vi "ep_Check Time Domain Parameters.vi"(5 "actual ranges [%]":dbl[](array[numeric]), 7 "ranges to calibrate [%]":dbl[](array[numeric]), 8 "error in (no error)":errorcluster, 9 "gains":dbl[][](array[numeric]), 10 "offsets":dbl[](array[numeric]), 11 "waveforms in":waveform(dbl)[](array[waveform])) -> (0 "error out":errorcluster)   [LabVIEW 2014, in "NI_EP_Power Quality.lvlib"]
uses:
  <vilib>/addons/Electrical Power/PQ/NI_EP_Power Quality.lvlib
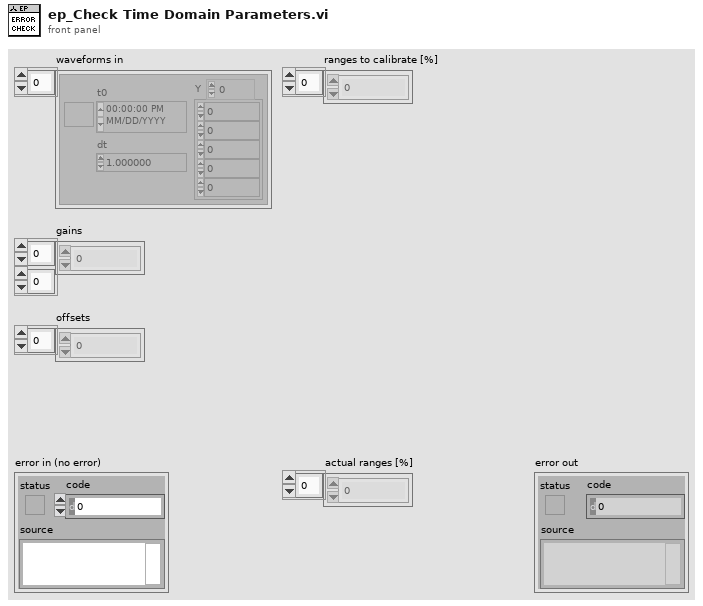
[diagram p1: front panel]
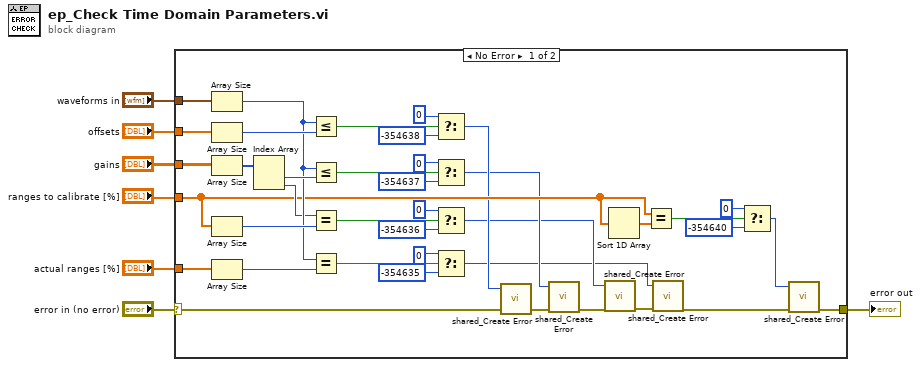
[diagram p0: block diagram]
diagram:
  n1 = case shown="No Error" "error in (no error)" {
    selector: "error in (no error)" -> [w8 w47]
    tunnel: "waveforms in" -> [w45 _]
    tunnel: "offsets" -> [w44 _]
    tunnel: "actual ranges [%]" -> [w43 _]
    tunnel: "gains" -> [w40 _]
    tunnel: "ranges to calibrate [%]" -> [w35 _]
    tunnel: [w9 w47] -> w2
    frame No Error {
      n2 = Array Size(array=w45) -> (size(s)=w37:i32)
      n3 = Array Size(array=w44) -> (size(s)=w46:i32)
      n4 = Array Size(array=w40) -> (size(s)=w39:i32[])
      n5 = Array Size(array=w35) -> (size(s)=w41:i32)
      n6 = Array Size(array=w43) -> (size(s)=w42:i32)
      n7 = Index Array(array=w39) -> (element #1=w38:i32, element #2=w36:i32)  [unwired: 2 in]
      n8 = Less Or Equal?(x=w37, y=w46) -> (x <= y?=w33:bool)
      n9 = Less Or Equal?(x=w37, y=w38) -> (x <= y?=w30:bool)
      n10 = Equal?(x=w36, y=w41) -> (x = y?=w31:bool)
      n11 = Equal?(x=w37, y=w42) -> (x = y?=w32:bool)
      n12 = Select(t=0 ("error code (0)"), s=w33, f=-354638 ("error code (0)")) -> (s? t:f=w24:i32)
      n13 = Select(t=0 ("error code (0)"), s=w30, f=-354637 ("error code (0)")) -> (s? t:f=w21:i32)
      n14 = Select(t=0 ("error code (0)"), s=w31, f=-354636 ("error code (0)")) -> (s? t:f=w18:i32)
      n15 = Select(t=0 ("error code (0)"), s=w32, f=-354635 ("error code (0)")) -> (s? t:f=w15:i32)
      n16 = call <vilib>:"shared_Create Error.vi"("error in (no error)"=w8, "error code (0)"=w24) -> ("error out"=w22:errorcluster)  [unwired: 9 in]
      n17 = call <vilib>:"shared_Create Error.vi"("error in (no error)"=w22, "error code (0)"=w21) -> ("error out"=w19:errorcluster)  [unwired: 9 in]
      n18 = call <vilib>:"shared_Create Error.vi"("error in (no error)"=w19, "error code (0)"=w18) -> ("error out"=w17:errorcluster)  [unwired: 9 in]
      n19 = Sort 1D Array(array=w35) -> (sorted array=w34:dbl[])
      n20 = Equal?(x=w35, y=w34) -> (x = y?=w13:bool)
      n21 = call <vilib>:"shared_Create Error.vi"("error in (no error)"=w17, "error code (0)"=w15) -> ("error out"=w11:errorcluster)  [unwired: 9 in]
      n22 = Select(t=0 ("error code (0)"), s=w13, f=-354640 ("error code (0)")) -> (s? t:f=w10:i32)
      n23 = call <vilib>:"shared_Create Error.vi"("error in (no error)"=w11, "error code (0)"=w10) -> ("error out"=w9:errorcluster)  [unwired: 9 in]
    }
    frame Error {
    }
  }
  "error out" <- w2
